vi "Get Most Recent Color Image16.vi"(0 "size":u32, 1 "blue":u16, 5 "algorithm":i32, 7 "red":u16, 9 "green":u16, 11 "error in (no error)":errorcluster) -> (3 "blue out":u16, 4 "function return":u32, 8 "red out":u16, 10 "green out":u16, 15 "error out":errorcluster)   [LabVIEW 2014, in "atmcd32d.lvlib"]
doc: "unsigned int WINAPI GetMostRecentColorImage16(unsigned long size, int algorithm, WORD * red, WORD * green, WORD * blue);"
uses:
  atmcd32d.lvlib
  atmcd32d.dll
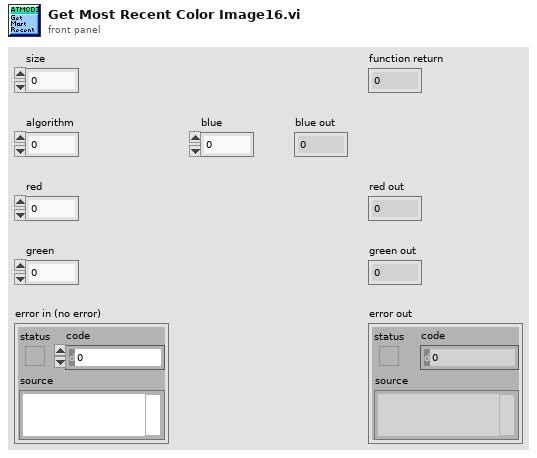
[diagram p1: front panel]
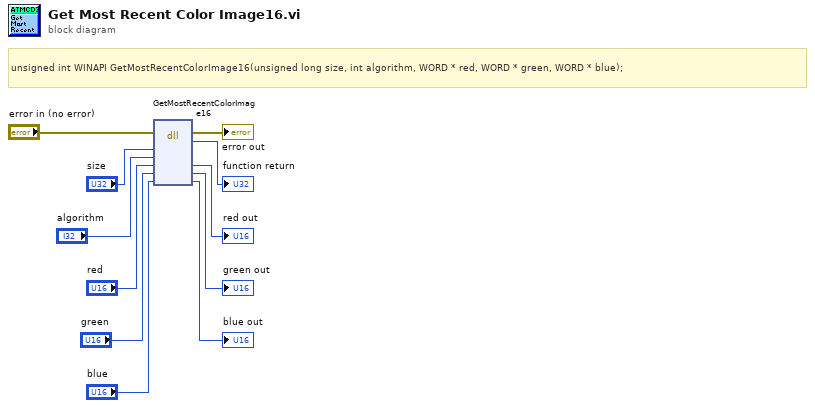
[diagram p0: block diagram]
diagram:
  # "unsigned int WINAPI GetMostRecentColorImage16(unsigned long size, int algorithm, WORD * red, WORD * green, WORD * blue);"
  n1 = dll-call lib="C:/Users/Bakir/Documents/Lambda2-Testing/lib/Andorlib/atmcd32d.*" fn="GetMostRecentColorImage16"(error in="error in (no error)", "size"="size", "algorithm"="algorithm", "red"="red", "green"="green", "blue"="blue") -> (error out=→"error out":errorcluster, →"function return":u32, "red"=→"red out":u16, "green"=→"green out":u16, "blue"=→"blue out":u16)  [unwired: 4 in, 1 out]
